vi "PXI-Compute Multiplier With Margin.vi"(7 "Mult In":dbl, 13 "margin (dB)":dbl=2.0) -> (8 "Mult Out":dbl)   [LabVIEW 2020]
uses:
  Utility VIs/Math VIs/dB to Linear (scalar).vi
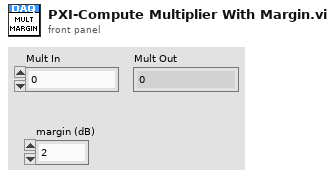
[diagram p1: front panel]
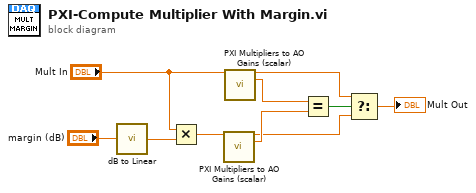
[diagram p0: block diagram]
diagram:
  n1 = call-poly "dB to Linear.vi"("dB"="margin (dB)") -> ("linear"=w9:dbl)
  n2 = Multiply(x="Mult In", y=w9) -> (x*y=w7:dbl)
  n3 = call "PXI Multipliers to AO Gains (scalar).vi"("Multiplier In"=w7) -> ("Multiplier Out"=w2:dbl, "Gain"=w6:dbl)  [unwired: 12 in, 1 out]
  n4 = call "PXI Multipliers to AO Gains (scalar).vi"("Multiplier In"="Mult In") -> ("Multiplier Out"=w3:dbl, "Gain"=w4:dbl)  [unwired: 12 in, 1 out]
  n5 = Equal?(x=w4, y=w6) -> (x = y?=w5:bool)
  n6 = Select(t=w3, s=w5, f=w2) -> (s? t:f=→"Mult Out":dbl)
